vi "Read Serial port.vi"(8 "error in (no error)":errorcluster, 11 "Motor-Serial in":refnum<class "Motor-Serial.lvclass">) -> (0 "error out":errorcluster, 2 "Serial port":refnum<visa-resource-name>, 3 "Motor-Serial out":refnum<class "Motor-Serial.lvclass">)   [LabVIEW 2013, in "PowderDeposition.lvlib" / "Motor-Serial.lvclass"]
uses:
  Motor-Serial.lvclass
  Motor-Serial.lvclass/Motor-Serial.ctl
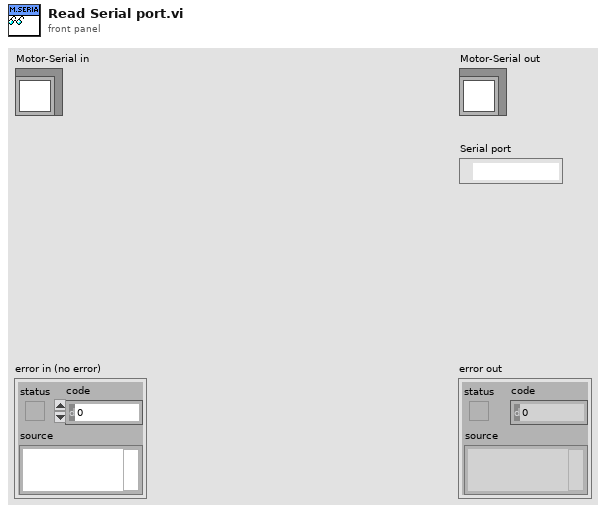
[diagram p1: front panel]
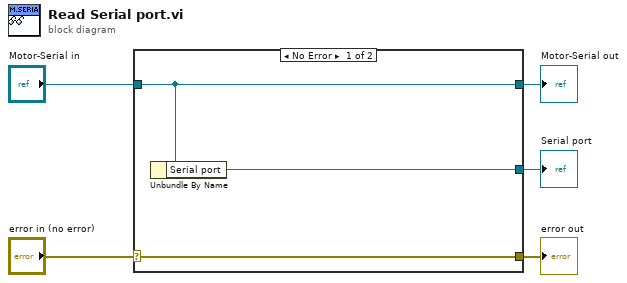
[diagram p0: block diagram]
diagram:
  n1 = case shown="No Error" "error in (no error)" {
    selector: "error in (no error)" -> [w8 w9]
    tunnel: [w8 w9] -> w4
    tunnel: [w7 w10] -> w2
    tunnel: "Motor-Serial in" -> [w7 w10]
    tunnel: [w6 _] -> w1
    frame No Error {
      n2 = Unbundle By Name(w7) -> ("Serial port"=w6:refnum<visa-resource-name>)
    }
    frame Error {
    }
  }
  "error out" <- w4
  "Motor-Serial out" <- w2
  "Serial port" <- w1
